vi "Pixel Location Global.vi"() -> ()   [LabVIEW 2013]
panel:
  in  "# of Frames to Average":u8
  in  "Avg Frame Count":u8
  in  "Y Resolution":u16=1088
  in  "X Resolution":u16=2040
  in  "Current Y Pixel Location":u16
  in  "Current X Pixel Location":u16
  # "For counting every third frame to process.\nNeed to reset if after"
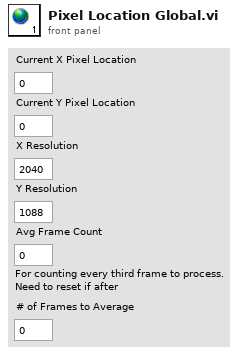
[diagram p1: front panel]
diagram:
